vi "Z900_navX_Internal_StartLoop.vi"(8 "error in (no error)":errorcluster, 11 "navX Device":T1={"Interface"={"Protocol"=enum."SERIAL", "Update Rate (4Hz-60Hz)"=4, "navX Open TypeDef"=variant}, "Notify Packet"=refnum, "Loop VI Refnum"=refnum} {"Interface"."Update Rate (4Hz-60Hz)" min=4 max=60 step=1}) -> (0 "error out":errorcluster, 3 "navX Device":T1={"Interface"={"Protocol"=enum."SERIAL", "Update Rate (4Hz-60Hz)"=4, "navX Open TypeDef"=variant}, "Notify Packet"=refnum, "Loop VI Refnum"=refnum} {"Interface"."Update Rate (4Hz-60Hz)" min=4 max=60 step=1})   [LabVIEW 2014, in "navX Library v2.lvlib"]
uses:
  navX Library v2.lvlib
  TypeDefs/Z900_navX_DeviceTypeDef.ctl
  TypeDefs/Z900_navX_ProtocolTypeDef.ctl
  TypeDefs/Z900_navX_NotifyPacketTypeDef.ctl
  TypeDefs/Z900_navX_ActionTypeDef.ctl
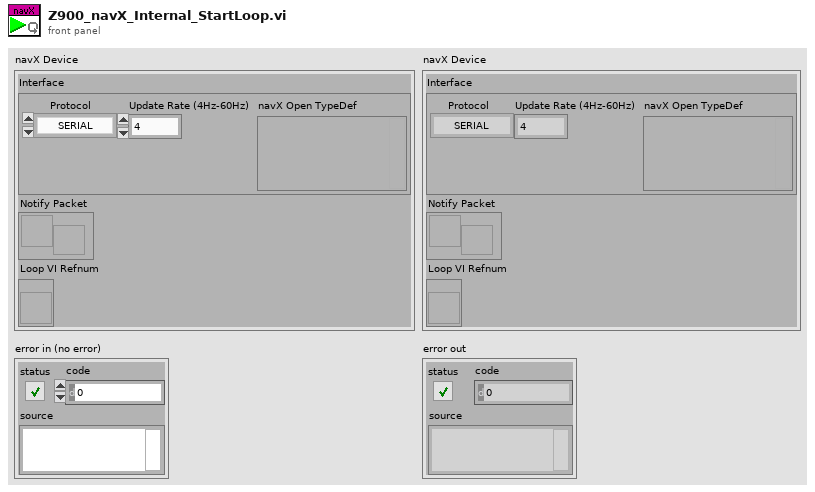
[diagram p1: front panel]
types:
  T1 = typedef "navX Library v2.lvlib/Z900_navX_DeviceTypeDef.ctl" = cluster{"Interface":cluster{"Protocol":T2, "Update Rate (4Hz-60Hz)":u8, "navX Open TypeDef":variant}, "Notify Packet":refnum<notifier>, "Loop VI Refnum":refnum<vi>}
  T2 = typedef "navX Library v2.lvlib/Z900_navX_ProtocolTypeDef.ctl" = enum16{"SERIAL", "I2C", "SPI"}
  T3 = typedef "navX Library v2.lvlib/Z900_navX_NotifyPacketTypeDef.ctl" = cluster{"navX Action":T4, "Data":variant}
  T4 = typedef "navX Library v2.lvlib/Z900_navX_ActionTypeDef.ctl" = enum16{"None", "Halt", "Zero-Yaw", "Update Serial Protocol"}
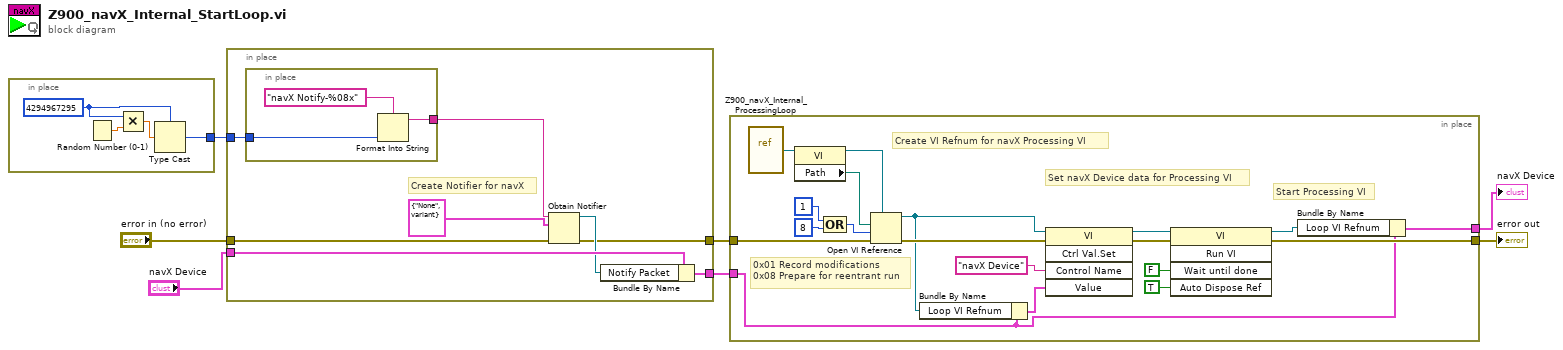
[diagram p0: block diagram]
diagram:
  n1 = in-place {
    in-place-border: [w8] -> w7
    w10 = u32 4294967295
    n2 = Random Number (0-1)() -> (number: 0 to 1=w11:dbl)
    n3 = Multiply(x=w10, y=w11) -> (x*y=w9:dbl)
    n4 = Type Cast(type=w10, x=w9) -> (*(type *) &x=w8:u32)
  }
  n5 = in-place {
    in-place-border: "navX Device" -> [w19]
    in-place-border: [w18] -> w3
    in-place-border: "error in (no error)" -> [w15]
    in-place-border: w7 -> [w13]
    in-place-border: [w12] -> w4
    # "Create Notifier for navX"
    n6 = in-place {
      in-place-border: [w21] -> w14
      in-place-border: w13 -> [w20]
      n7 = Format Into String(format string="navX Notify-%08x" ("name (unnamed)"), w20) -> (resulting string=w21:string)  [unwired: 2 in, 1 out]
    }
    n8 = Obtain Notifier(name (unnamed)=w14, notification data type=T3 {"navX Action"=enum."None", "Data"=variant} ("navX Notify Packet"), error in (no error)=w15) -> (notifier out=w17:refnum<notifier>, error out=w12:errorcluster)  [unwired: 1 in, 1 out]
    n9 = Bundle By Name(cluster=w19, "Notify Packet"=w17) -> (w18:T1)
  }
  n10 = in-place {
    in-place-border: w4 -> [w41]
    in-place-border: [w39] -> w2
    in-place-border: [w40] -> w1
    in-place-border: w3 -> [w38]
    # "0x01 Record modifications\n0x08 Prepare for reentrant run"
    # "Start Processing VI"
    # "Set navX Device data for Processing VI"
    # "Create VI Refnum for navX Processing VI"
    n11 = vi-ref "Z900_navX_Internal_ProcessingLoop.vi"() -> (w32:refnum<vi>)
    n12 = property class="VI"(reference=w32) -> (reference out=w37:refnum<vi>, "Path"=w36:path)  [unwired: 1 in, 1 out]
    n13 = Compound Arithmetic op=OR(1 ("value"), 8) -> (w35:i32)
    n14 = Open VI Reference(type specifier VI Refnum (for type only)=w37, vi path=w36, options=w35, error in (no error)=w41) -> (vi reference=w29:refnum<vi>, error out=w30:errorcluster)  [unwired: 2 in]
    n15 = Bundle By Name(cluster=w38, "Loop VI Refnum"=w29) -> (w28:T1)
    n16 = invoke class="VI" method="Ctrl Val.Set"(reference=w29, error in=w30, "Control Name"="navX Device" ("format string"), "Value"=w28) -> (reference out=w25:refnum<vi>, error out=w24:errorcluster)  [unwired: 1 in, 3 out]
    n17 = invoke class="VI" method="Run VI"(reference=w25, error in=w24, "Wait until done"=FALSE ("Wait Until Done"), "Auto Dispose Ref"=TRUE ("Auto Dispose Reference")) -> (reference out=w23:refnum<vi>, error out=w40:errorcluster)  [unwired: 1 in, 3 out]
    n18 = Bundle By Name(cluster=w38, "Loop VI Refnum"=w23) -> (w39:T1)
  }
  "navX Device" <- w2
  "error out" <- w1
